vi "RSNRPZ Set Averaging State.vi"(8 "error in (no error)":errorcluster, 9 "Averaging (On)":bool=TRUE, 10 "Channel (1)":i32=1, 11 "VISA session":refnum<visa-resource-name> caption="VISA resource name") -> (0 "error out":errorcluster, 3 "dup VISA session":refnum<visa-resource-name> caption="VISA resource name")   [LabVIEW 2010]
doc: "This VI switches the filter function of a sensor on or off. When the filter is switched on, the number of measured values set with RSNRPZ Set Averaging Count.vi is averaged. This reduces the effect of noise so that more reliable results are obtained.\n\nRemote-control command(s):\nSENS:AVER:STAT ON | OFF"
uses:
  rsnrpz_32.dll
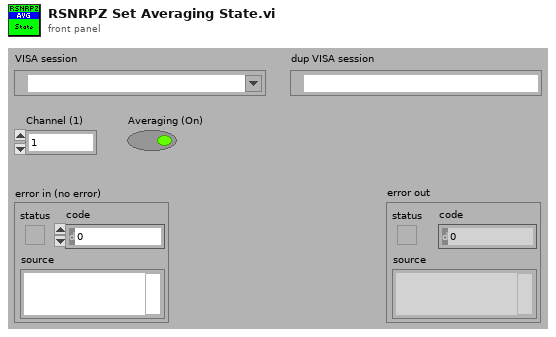
[diagram p1: front panel]
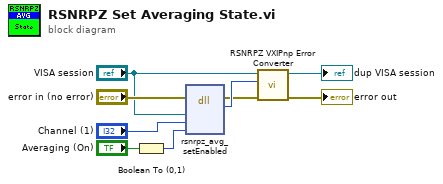
[diagram p0: block diagram]
diagram:
  n1 = Boolean To (0,1)(Boolean="Averaging (On)") -> (0, 1=w6:i16)
  n2 = dll-call lib="rsnrpz_32.dll" fn="rsnrpz_avg_setEnabled"(error in="error in (no error)", "VISA Session"="VISA session", "Channel"="Channel (1)", "Averaging"=w6) -> (error out=w5:errorcluster, "Status"=w8:i32)  [unwired: 5 in, 1 out]
  n3 = call <instrlib>:"RSNRPZ VXIPnp Error Converter.vi"("error in"=w5, "VXIPnp error code"=w8, "VISA session"="VISA session") -> ("error out"=→"error out":errorcluster, "dup VISA session"=→"dup VISA session":refnum<visa-resource-name>)  [unwired: 7 in]
